vi "GST-CCD Grab.vi"(8 "error in (no error)":errorcluster caption="错误输入（无错误）", 9 "相机选择":enum16{"Cam0", "Cam1"}(ring), 11 "曝光":i64) -> (0 "error out":errorcluster caption="错误输出", 2 "Image":T2(plugin-control), 3 "Session Out":T1 caption="CCD1 Session Out")   [LabVIEW 2017]
uses:
  <resource>/objmgr/imaqdx.rc
  <vilib>/vision/driver/NI_Vision_Acquisition_Software.lvlib
  <vilib>/vision/driver/IMAQdx.llb/IMAQdx Buffer Number Mode.ctl
  <vilib>/vision/driver/IMAQdx.llb/IMAQdx Camera Control Mode.ctl
  <vilib>/vision/driver/IMAQdx.llb/IMAQdx Acquisition Mode.ctl
  <vilib>/userdefined/High Color/IMAQdx.ctl
  <vilib>/vision/NI_Vision_Development_Module.lvlib
  Global System.vi
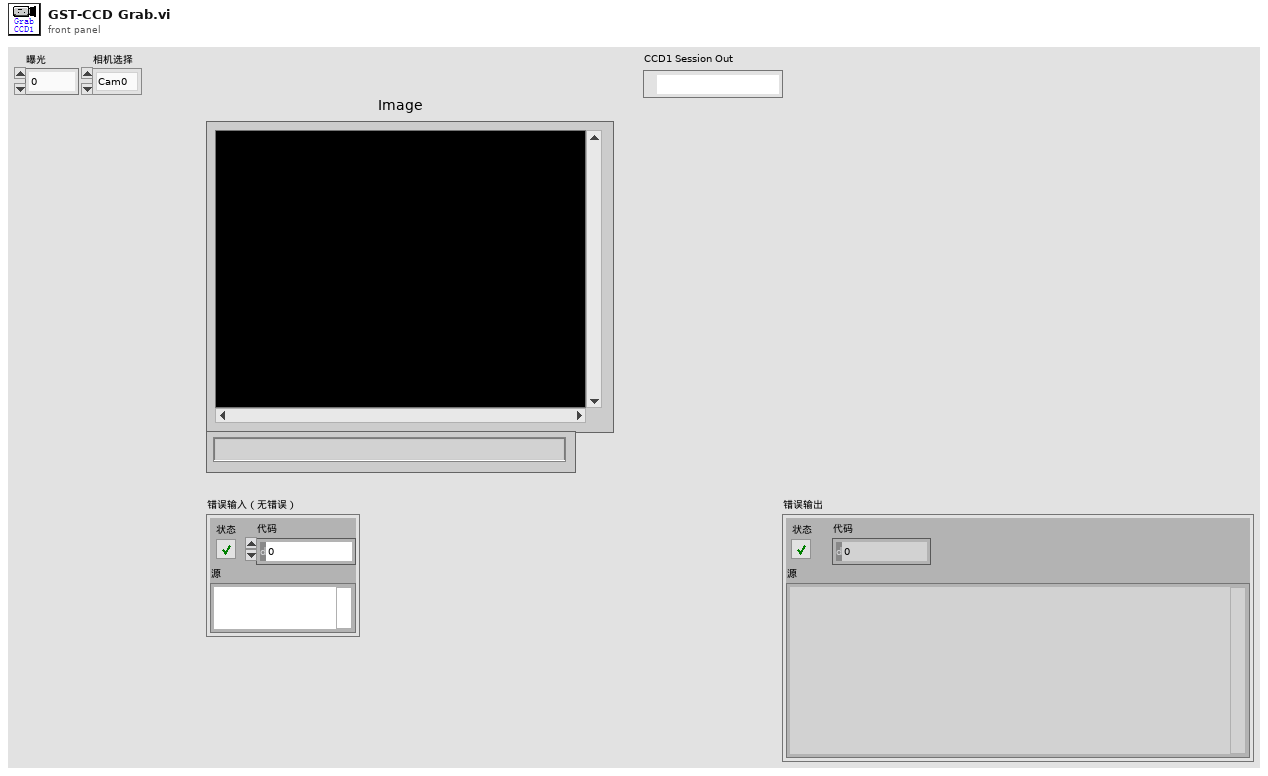
[diagram p1: front panel]
types:
  T1 = typedef "IMAQdx.ctl" = refnum<k21>
  T2 = typedef "IMAQ Image.ctl" = refnum<image>
  T3 = typedef "Image Type" = u32
  T4 = typedef "NI_Vision_Acquisition_Software.lvlib/IMAQdx Buffer Number Mode.ctl" = enum32{"Next", "Last", "Buffer Number", "Every", "Last New"}
  T5 = typedef "NI_Vision_Acquisition_Software.lvlib/IMAQdx Acquisition Mode.ctl" = enum32{"One Shot", "Continuous"}
  T6 = typedef "NI_Vision_Acquisition_Software.lvlib/IMAQdx Camera Control Mode.ctl" = enum32{"Controller", "Listener"}
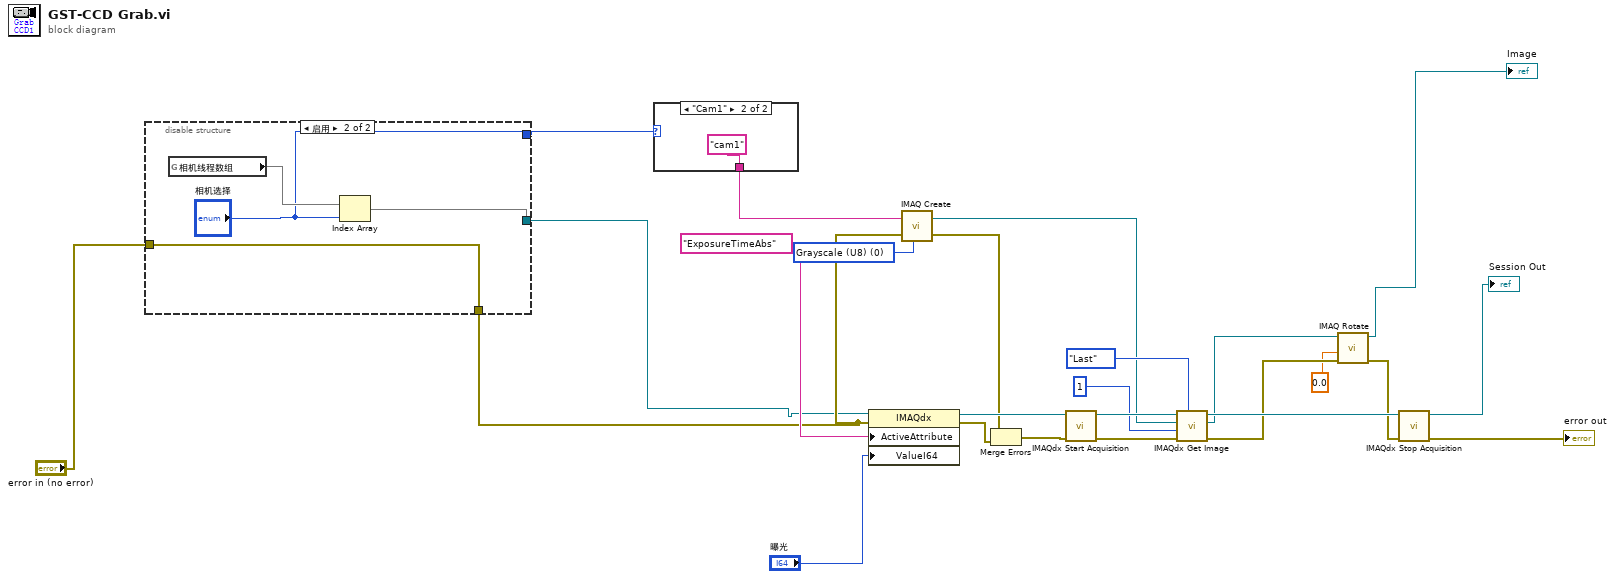
[diagram p0: block diagram]
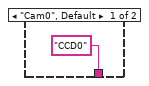
[diagram p2: hidden frame]
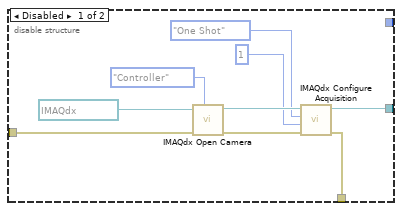
[diagram p3: hidden frame]
diagram:
  w1 = T3 0 items=["Grayscale (U8)", "Grayscale (I16)", "Grayscale (SGL)", "Complex (CSG)", "RGB (U32)", "HSL (U32)", "RGB (U64)", "Grayscale (U16)"] ("Image Type")
  n1 = disable-structure shown="启用" {
    disable-tunnel: "error in (no error)" -> [w28 w38]
    disable-tunnel: [w27 w38] -> w10
    disable-tunnel: [w26 w36] -> w9
    disable-tunnel: [_ "相机选择"] -> w3
    frame Disabled {
      n2 = call <vilib>:"IMAQdx Open Camera.vi"("Camera Control Mode"=IMAQdx_Camera_Control_Mode."Controller", "error in"=w28, "Session In"=T1 "acA2500-14gm") -> ("error out"=w29:errorcluster, "Session Out"=w33:T1)  [unwired: 7 in]
      n3 = call <vilib>:"IMAQdx Configure Acquisition.vi"("error in"=w29, "Number of Buffers"=u32 1, "Continuous?"=IMAQdx_Acquisition_Mode."One Shot", "Session In"=w33) -> ("error out"=w27:errorcluster, "Session Out"=w26:T1)  [unwired: 6 in]
    }
    frame Enabled {
      n4 = global read "Global System.vi" "相机线程数组"() -> (w37)
      n5 = Index Array(array=w37, index="相机选择") -> (element=w36)
    }
  }
  n6 = case shown="\"Cam1\"" w3 {
    tunnel: ["CCD0" ("Image Name") "cam1" ("Image Name")] -> w2
    frame "Cam0", Default {
    }
    frame "Cam1" {
    }
  }
  n7 = property class="IMAQdx"(reference=w9, error in=w10, "ActiveAttribute"="ExposureTimeAbs", "ValueI64"="曝光") -> (reference out=w24:T1, error out=w15:errorcluster)
  n8 = call "IMAQ Create"("Image Name"=w2, "Image Type"=w1, "error in (no error)"=w10) -> ("New Image"=w13:T2, "error out"=w16:errorcluster)  [unwired: 2 in]
  n9 = Merge Errors(w16, w15) -> (w14:errorcluster)
  n10 = call <vilib>:"IMAQdx Start Acquisition.vi"("error in"=w14, "Session In"=w24) -> ("error out"=w22:errorcluster, "Session Out"=w23:T1)  [unwired: 8 in]
  n11 = call <vilib>:"IMAQdx Get Image.vi"("Buffer Number Mode (Next)"=IMAQdx_Buffer_Number_Mode."Last", "error in"=w22, "Buffer Number In"=u32 1, "Image In"=w13, "Session In"=w23) -> ("error out"=w7:errorcluster, "Image Out"=w8:T2, "Session Out"=w19:T1)  [unwired: 3 in, 1 out]
  n12 = call "IMAQ Rotate"("error in (no error)"=w7, "Angle (degrees)"=sgl 0.0, "Image Src"=w8) -> ("error out"=w6:errorcluster, "Image Dst Out"=→"Image":T2)  [unwired: 7 in]
  n13 = call <vilib>:"IMAQdx Stop Acquisition.vi"("error in"=w6, "Session In"=w19) -> ("error out"=→"error out":errorcluster, "Session Out"=→"Session Out":T1)  [unwired: 8 in]
